vi "Finish.vi"   [LabVIEW 2014]
doc: "This VI is called just before exiting. It is expected to close I/O refnum, save collected data, etc."
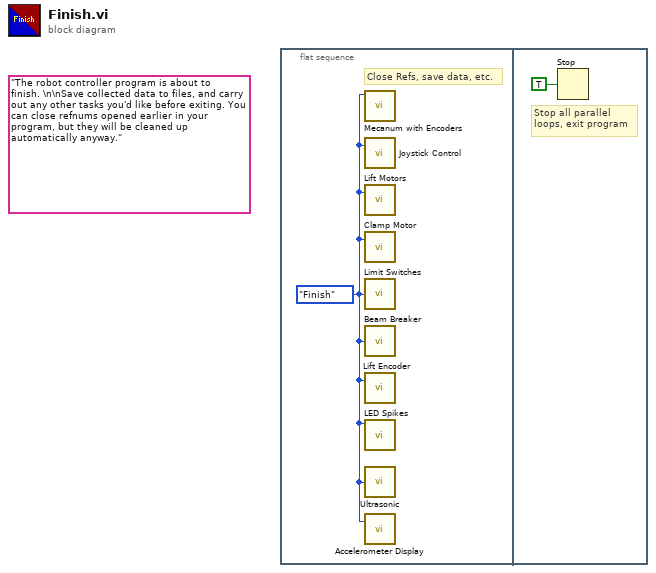
[diagram p0: block diagram]
diagram:
  (unwired) "The robot controller program is about to finish. \n\nSave collected data to files, and carry out any other tasks you'd like before exiting. You can close refnums opened earlier in your program, but they will be cleaned up automatically anyway."
  n1 = flat-sequence {
    frame #0 {
      w1 = enum16{"Start", "Run", "Finish"}."Finish" ("State Control")
      # "Close Refs, save data, etc."
      n2 = call "Mecanum with Encoders.vi"("Mode"=w1) -> ()  [unwired: 9 in, 1 out]
      n3 = call "Joystick Control.vi"("Mode"=w1) -> ()  [unwired: 1 in, 1 out]
      n4 = call "Lift Motors.vi"("Mode"=w1) -> ()  [unwired: 2 in]
      n5 = call "Clamp Motor.vi"("Mode"=w1) -> ()  [unwired: 2 in]
      n6 = call "Limit Switches.vi"("Mode"=w1) -> ()  [unwired: 1 out]
      n7 = call "Beam Breaker.vi"("Mode"=w1) -> ()  [unwired: 1 in, 1 out]
      n8 = call "Lift Encoder.vi"("Mode"=w1) -> ()  [unwired: 1 in, 1 out]
      n9 = call "LED Spikes.vi"("Mode"=w1) -> ()  [unwired: 3 in]
      n10 = call "Ultrasonic.vi"("Mode"=w1) -> ()  [unwired: 1 out]
      n11 = call "Accelerometer Display.vi"("Mode"=w1) -> ()  [unwired: 1 in, 1 out]
    }
    frame #1 {
      # "Stop all parallel\nloops, exit program"
      n12 = Stop(stop? (T)=TRUE ("Quit")) -> ()
    }
  }
